vi "Test - Compute Xi.vi"() -> ()   [LabVIEW 2014, in "HMM.lvlib"]
uses:
  HMM.lvlib
panel:
  out "Xi 2":dbl[][][](array[numeric])
  out "Xi":dbl[][][](array[numeric])
  in  "O Observed Sequence":i32[](array[numeric])
  in  "HMM Cluster":T1
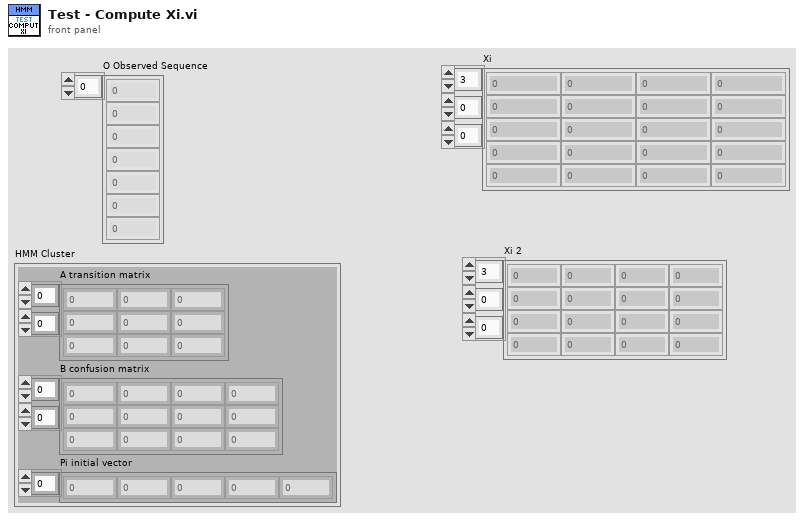
[diagram p1: front panel]
types:
  T1 = cluster{"A transition matrix":dbl[][], "B confusion matrix":dbl[][], "Pi initial vector":dbl[]}
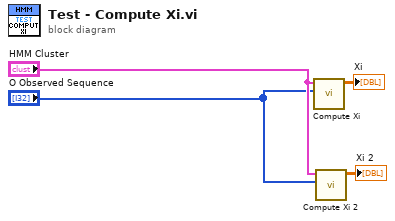
[diagram p0: block diagram]
diagram:
  n1 = call "Compute Xi.vi"("Observed sequence O"="O Observed Sequence", "HMM Cluster"="HMM Cluster") -> ("Xi"=→"Xi":dbl[][][])  [unwired: 9 in]
  n2 = call "Compute Xi 2.vi"("Observed sequence O"="O Observed Sequence", "HMM Cluster"="HMM Cluster") -> ("Xi"=→"Xi 2":dbl[][][])  [unwired: 9 in]
